vi "DO Main.vi"(8 "error In":errorcluster, 11 "All Queue":T1) -> (0 "error out 2":errorcluster)   [LabVIEW 2022 SP3]
uses:
  Controls/All Queue Ref.ctl
  Controls/ALL Health.ctl
  <vilib>/DAQmx/write.llb/DAQmx Write (Digital 1D Bool NChan 1Samp 1Line).vi
  6D_Global.vi
  <vilib>/DAQmx/create/channels.llb/DAQmx Create Channel (DO-Digital Output).vi
  <vilib>/DAQmx/miscellaneous.llb/DAQmx Fill In Error Info.vi
panel:
  in  "DO  Configuration":cluster{"NAME":string, "lines":tag}[](array[cluster])=[{"NAME"="GD COM", "lines"="cDAQ9185-1E540F5Mod1/port0/line0"}, {"NAME"="Motor Command", "lines"="cDAQ9185-1E540F5Mod1/port0/line1"}]
  out "Loop Rate 2":u32
  out "DO wave":waveform(dbl)[](array[waveform])
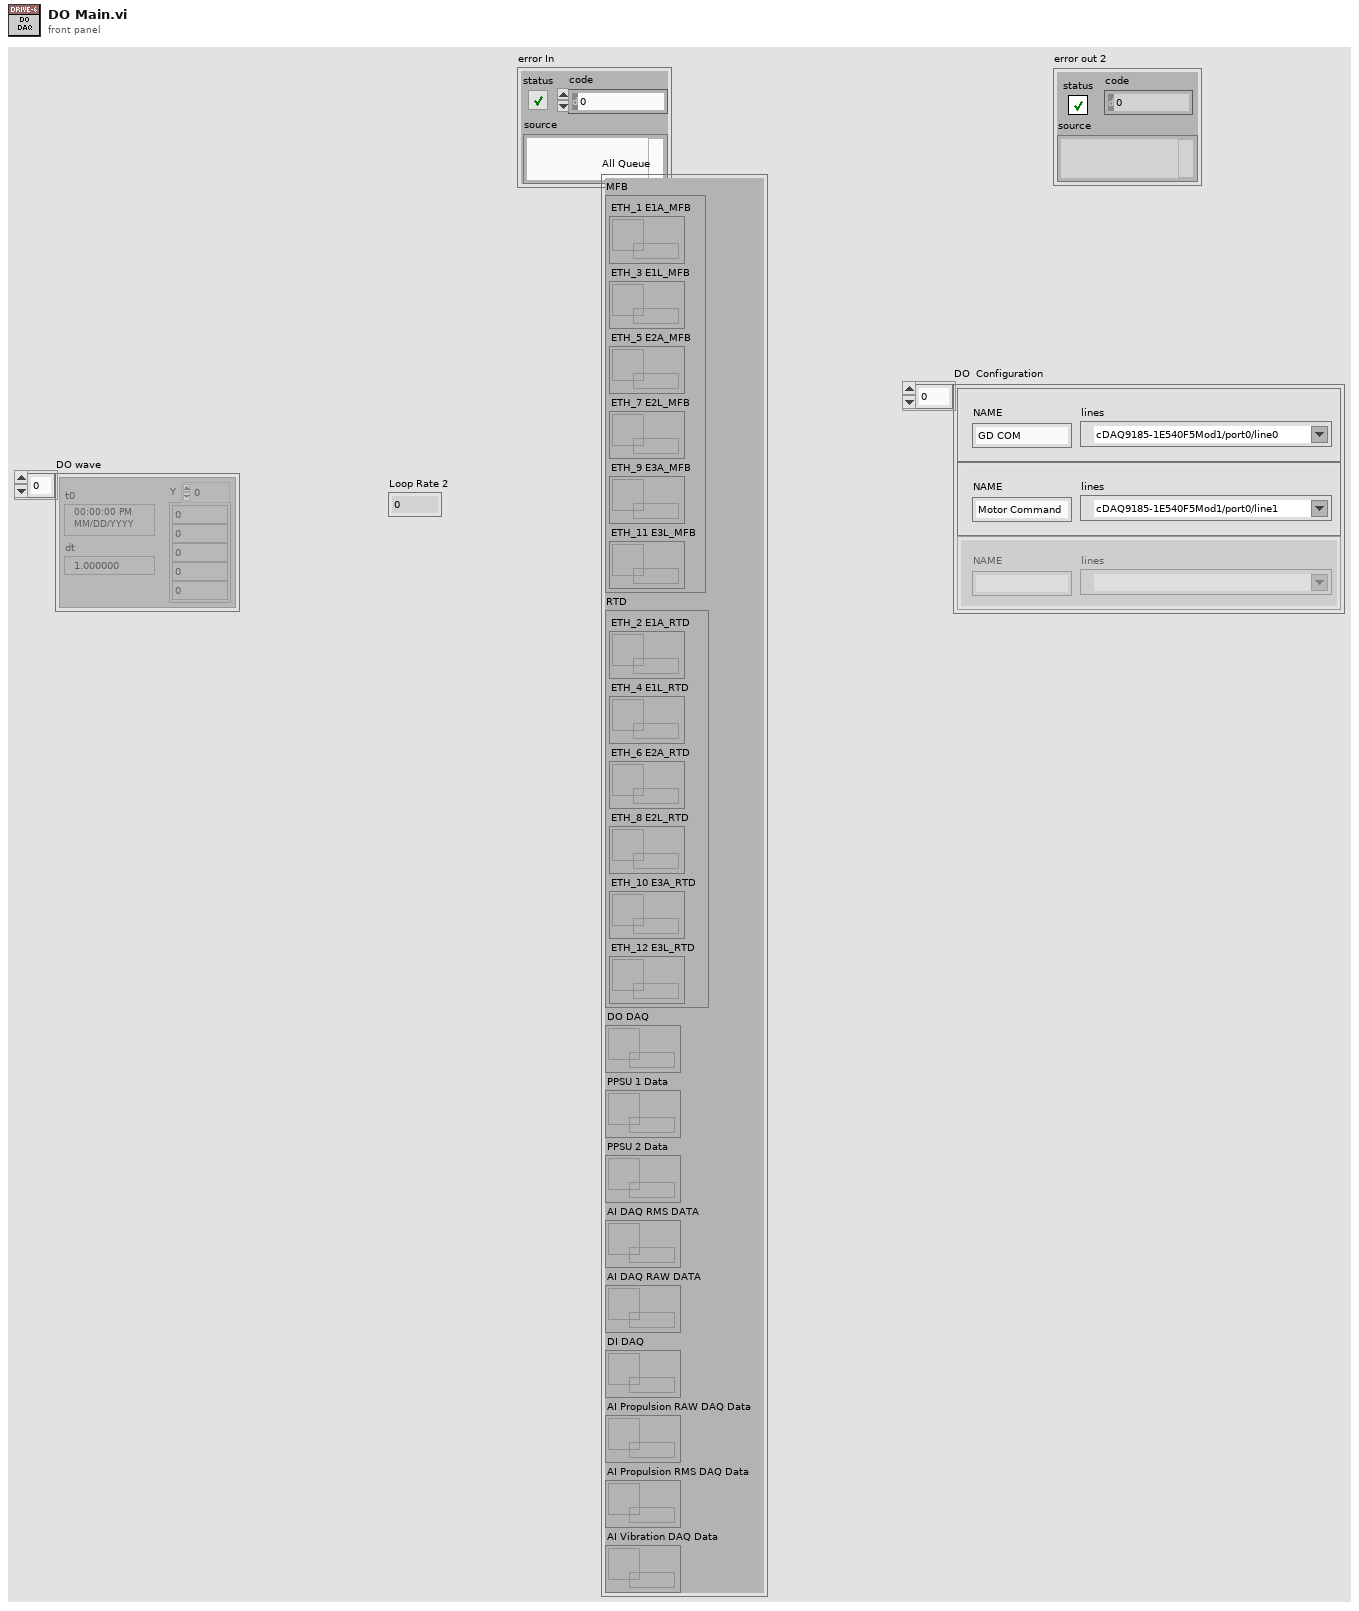
[diagram p1: front panel]
types:
  T1 = typedef "All Queue Ref.ctl" = cluster{"MFB":cluster{"ETH_1 E1A_MFB":refnum<queue>, "ETH_3 E1L_MFB":refnum<queue>, "ETH_5 E2A_MFB":refnum<queue>, "ETH_7 E2L_MFB":refnum<queue>, "ETH_9 E3A_MFB":refnum<queue>, "ETH_11 E3L_MFB":refnum<queue>}, "RTD":cluster{"ETH_2 E1A_RTD ":refnum<queue>, "ETH_4 E1L_RTD ":refnum<queue>, "ETH_6 E2A_RTD ":refnum<queue>, "ETH_8 E2L_RTD ":refnum<queue>, "ETH_10 E3A_RTD ":refnum<queue>, "ETH_12 E3L_RTD ":refnum<queue>}, "DO DAQ":refnum<queue>, "PPSU 1 Data":refnum<queue>, "PPSU 2 Data":refnum<queue>, "AI DAQ RMS DATA":refnum<queue>, "AI DAQ RAW DATA":refnum<queue>, "DI DAQ":refnum<queue>, "AI Propulsion RAW DAQ Data":refnum<queue>, "AI Propulsion RMS DAQ Data":refnum<queue>, "AI Vibration DAQ Data":refnum<queue>}
  T2 = enum16{"Init", "Read 'All'", "Read 'n'", "Read '1'", "Write '1'", "Write 'n'", "Write 'All'"}
  T3 = typedef "ALL Health.ctl" = enum16{"AI HS", "AI Vibration HS", "AI Propulsion HS", "DO HS", "Datalog HS", "PPSU HS", "ETH_1 DAQ", "ETH_1 RTD", "ETH_2 DAQ", "ETH_2 RTD", "ETH_5 RTD"}
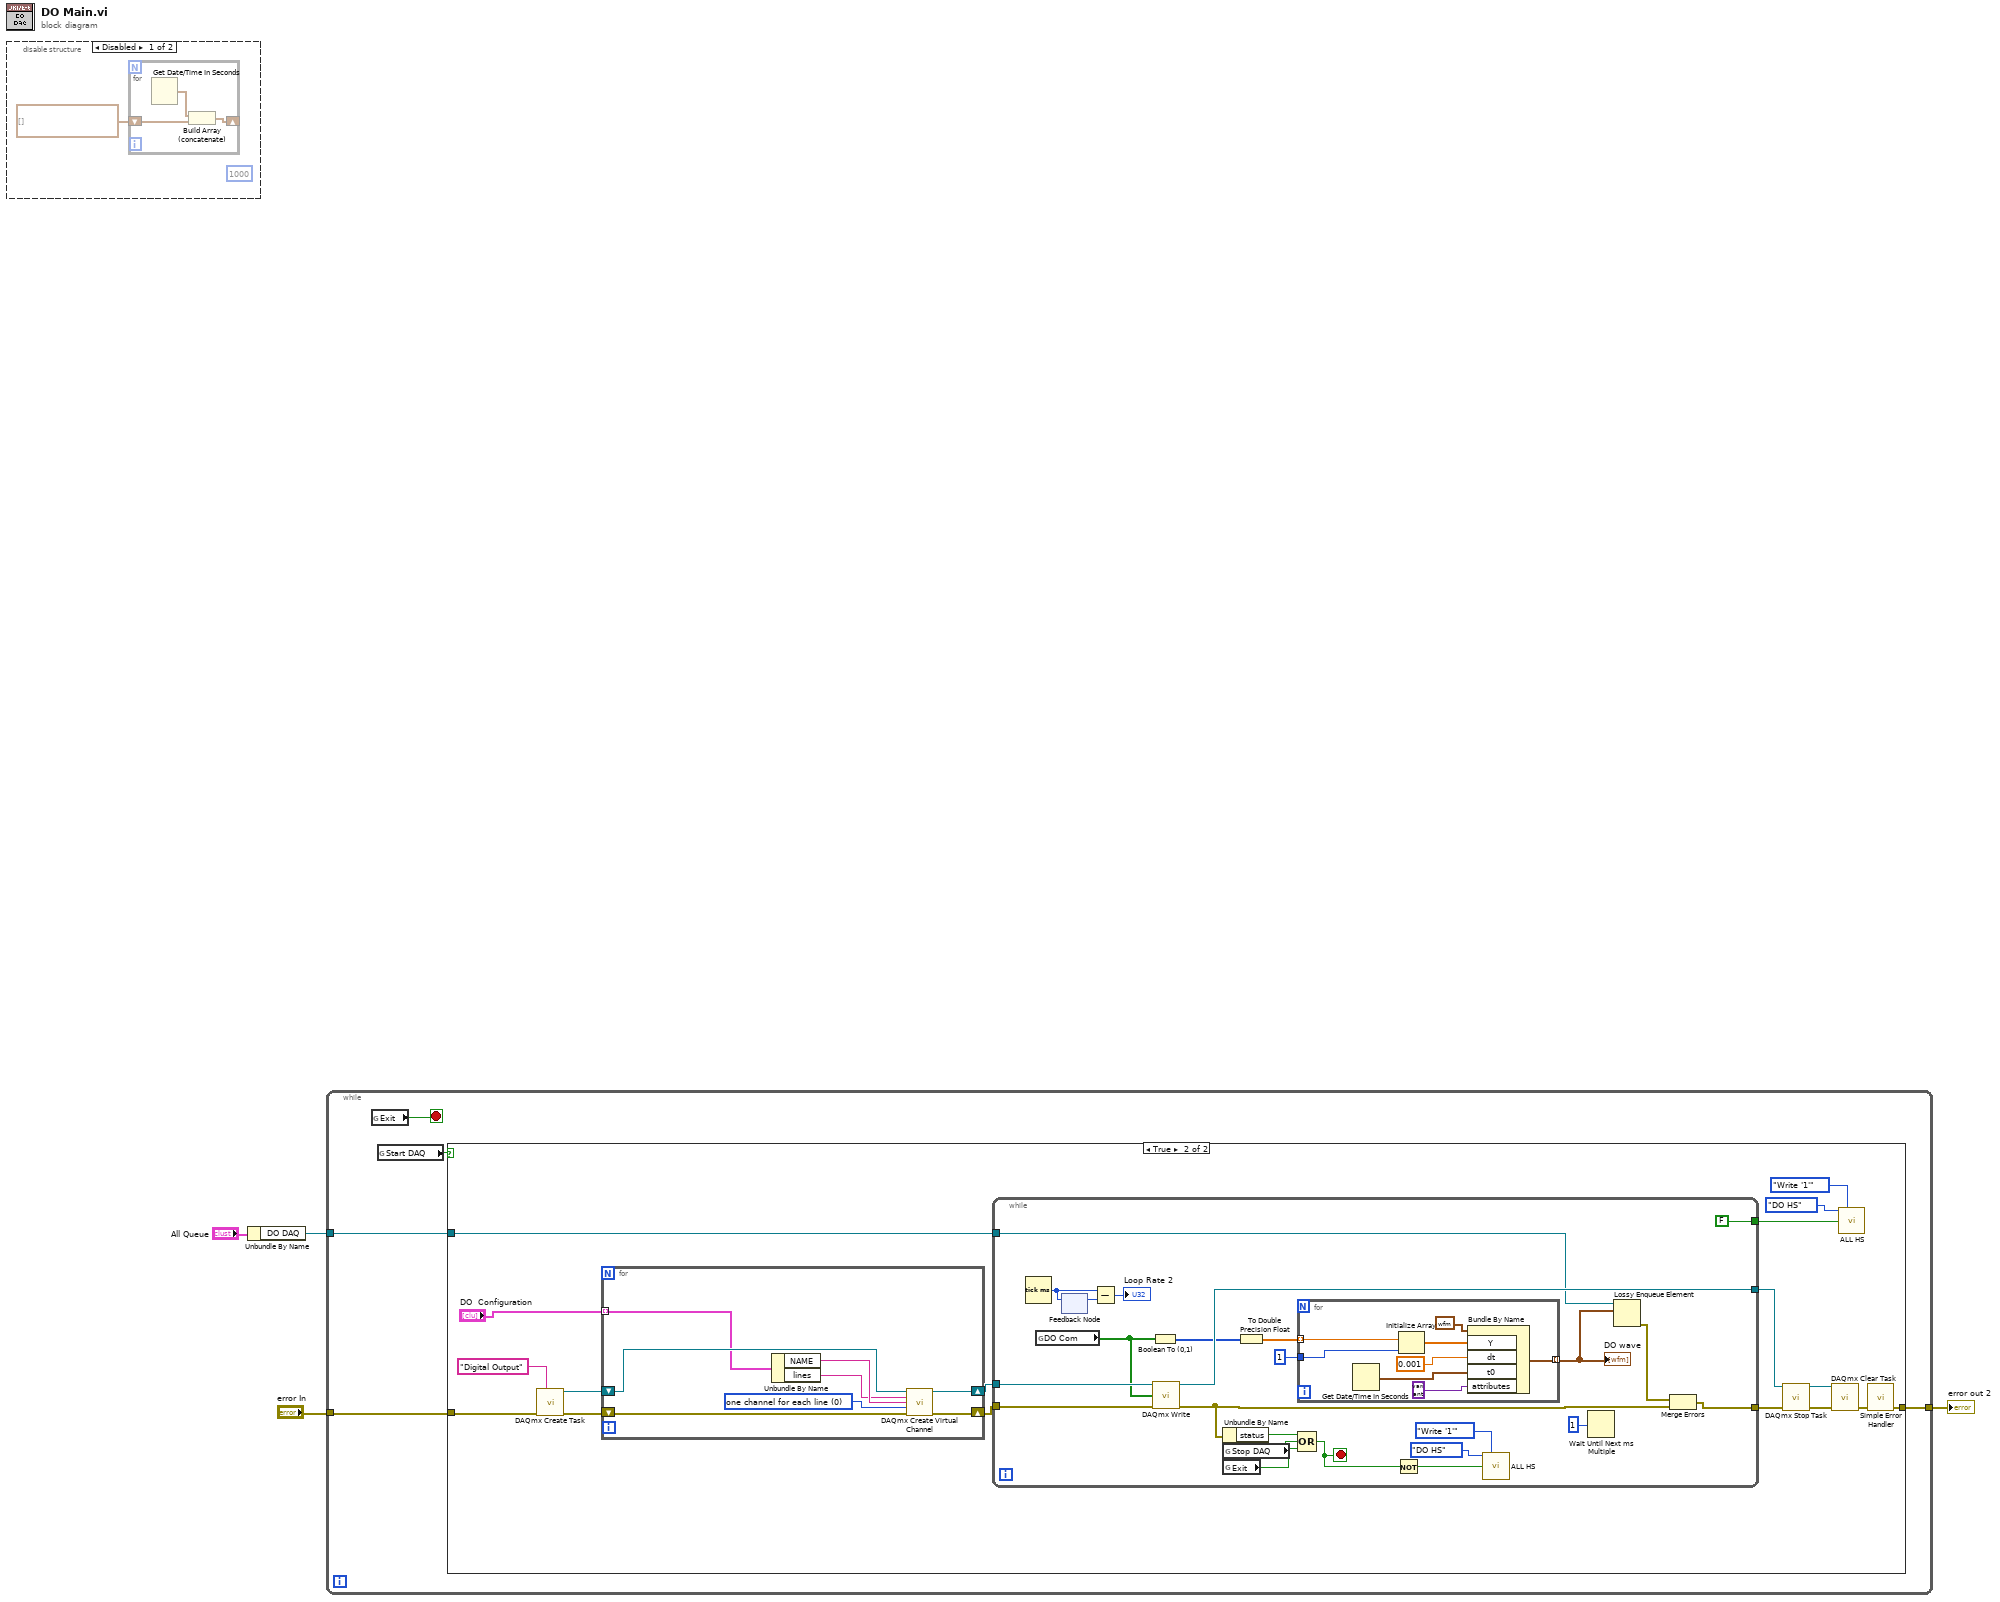
[diagram p0: block diagram]
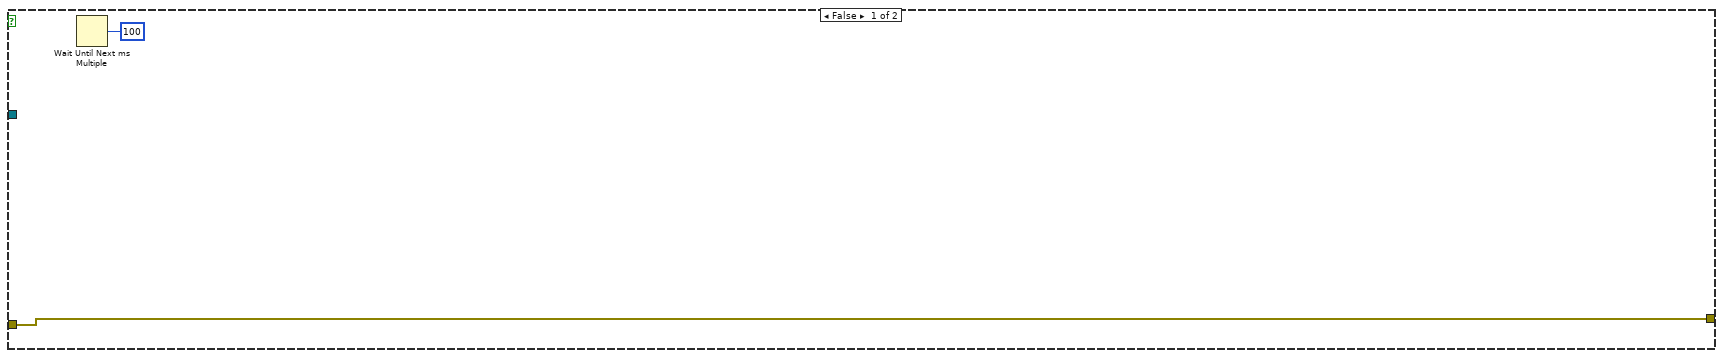
[diagram p2: hidden frame]
diagram:
  n1 = disable-structure shown="Disabled" {
    frame Disabled {
      (unwired) 1000
      n2 = for {
        shift-right: [w7] -> _
        shift-left: timestamp[] [] -> [w6]
        n3 = Get Date/Time In Seconds() -> (seconds since 1Jan1904=w8:timestamp)
        n4 = Build Array (concatenate)(w8, w6) -> (w7:timestamp[])
      }
    }
    frame Enabled {
    }
  }
  n5 = Unbundle By Name("All Queue") -> ("DO DAQ"=w1:refnum<queue>)
  n6 = while {
    tunnel: [w13] -> w4
    tunnel: "error In" -> [w12]
    tunnel: w1 -> [w9]
    stop <- w11 stop-if-true
    n7 = global read "6D_Global.vi" "Exit"() -> (w11:bool)
    n8 = global read "6D_Global.vi" "Start DAQ"() -> (w10:bool)
    n9 = case shown="True" w10 {
      tunnel: [w14 w25] -> w13
      tunnel: w12 -> [w14 w23]
      tunnel: w9 -> [_ w20]
      frame False {
        n10 = Wait Until Next ms Multiple(millisecond multiple=u32 100) -> ()  [unwired: 1 out]
      }
      frame True {
        n11 = call <vilib>:"DAQmx Create Task.vi"("new task name"="Digital Output", "error in"=w23) -> ("task out"=w22:refnum<k21>, "error out"=w24:errorcluster)  [unwired: 12 in]
        n12 = for {
          shift-right: [w69] -> w27
          shift-left: w22 -> [w72]
          shift-right: [w68] -> w26
          shift-left: w24 -> [w71]
          tunnel: "DO  Configuration" -> [w65] mode=indexing
          w70 = 0 items=["one channel for each line", "one channel for all lines"] ("line grouping")
          n13 = Unbundle By Name(w65) -> ("NAME"=w67:string, "lines"=w66:tag)
          n14 = call-poly <vilib>:"DAQmx Create Virtual Channel.vi"("task in"=w72, "lines"=w66, "name to assign"=w67, "line grouping"=w70, "error in"=w71) -> ("task out"=w69:refnum<k21>, "error out"=w68:errorcluster)  [unwired: 9 in]
        }
        n15 = while {
          tunnel: w27 -> [w56]
          tunnel: w26 -> [w55]
          tunnel: [w54] -> w28
          tunnel: [w37] -> w32
          tunnel: [FALSE ("DO Health")] -> w17
          tunnel: w20 -> [w40]
          stop <- w52 stop-if-true
          n16 = Tick Count (ms)() -> (millisecond timer value=w51:u32)
          n17 = global read "6D_Global.vi" "DO Com"() -> (w43:bool[])
          n18 = feedback #1() -> (w50:u32)  [unwired: 1 in]
          n19 = feedback-in #1(w51) -> ()
          n20 = Subtract(x=w51, y=w50) -> (x-y=→"Loop Rate 2":u32)
          n21 = Boolean To (0,1)(Boolean=w43) -> (0, 1=w45:i16[])
          n22 = call-poly <vilib>:"DAQmx Write.vi"("task/channels in"=w56, "data"=w43, "error in"=w55) -> ("task out"=w54:refnum<k21>, "error out"=w38:errorcluster)  [unwired: 10 in, 1 out]
          n23 = Unbundle By Name(w38) -> ("status"=w53:bool)
          n24 = global read "6D_Global.vi" "Stop DAQ"() -> (w41:bool)
          n25 = global read "6D_Global.vi" "Exit"() -> (w42:bool)
          n26 = To Double Precision Float(number=w45) -> (double precision float=w47:dbl[])
          n27 = for {
            tunnel: w47 -> [w64] mode=indexing
            tunnel: 1 ("dimension size") -> [w63]
            tunnel: [w59] -> w39 mode=indexing
            n28 = Get Date/Time In Seconds() -> (seconds since 1Jan1904=w57:timestamp)
            n29 = Initialize Array(w64, w63) -> (w62:dbl[])
            n30 = Bundle By Name(cluster=waveform(dbl) {"t0"=timestamp(0 s since 1904-01-01), "dt"=1.0, "Y"=[]} ("waveform"), "Y"=w62, "dt"=0.001, "t0"=w57, "attributes"=variant) -> (w59:waveform(dbl))
          }
          "DO wave" <- w39
          n31 = Compound Arithmetic op=OR(w53, w41, w42) -> (w52:bool)
          n32 = Not(x=w52) -> (.not. x?=w34:bool)
          n33 = call "ALL HS.vi"("Loop"=ALL_Health."DO HS", "Option"=T2."Write '1'", "Status"=w34) -> ()  [unwired: 10 in, 3 out]
          n34 = Wait Until Next ms Multiple(millisecond multiple=u32 1) -> ()  [unwired: 1 out]
          n35 = Lossy Enqueue Element(queue=w40, element=w39) -> (error out=w36:errorcluster)  [unwired: 1 in, 3 out]
          n36 = Merge Errors(w36, w38) -> (w37:errorcluster)
        }
        n37 = call <vilib>:"DAQmx Stop Task.vi"("task/channels in"=w28, "error in"=w32) -> ("task out"=w31:refnum<k21>, "error out"=w30:errorcluster)  [unwired: 12 in]
        n38 = call <vilib>:"DAQmx Clear Task.vi"("task in"=w31, "error in"=w30) -> ("error out"=w29:errorcluster)  [unwired: 13 in]
        n39 = call "ALL HS.vi"("Loop"=ALL_Health."DO HS", "Option"=T2."Write '1'", "Status"=w17) -> ()  [unwired: 10 in, 3 out]
        n40 = call <vilib>:"Simple Error Handler.vi"("error in (no error)"=w29) -> ("error out"=w25:errorcluster)  [unwired: 4 in, 4 out]
      }
    }
  }
  "error out 2" <- w4
